vi "End Game.vi"(8 "error in (no error)":errorcluster, 11 "Game in":refnum<class "Game.lvclass">) -> (0 "error out":errorcluster, 3 "Game out":refnum<class "Game.lvclass">)   [LabVIEW 2020, in "SquareBattle.lvlib" / "Game.lvclass"]
uses:
  Game.lvclass
  Game.lvclass/Game.ctl
  Map/Map.lvclass
  Team/Team.lvclass
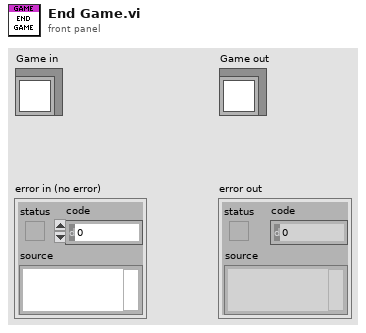
[diagram p1: front panel]
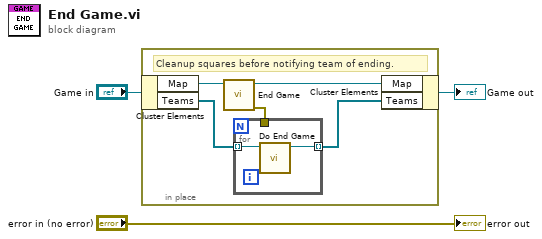
[diagram p0: block diagram]
diagram:
  n1 = in-place {
    # "Cleanup squares before notifying team of ending."
    n2 = in-place-cluster #1("Game in") -> ("Map"=w8:refnum<class "Map.lvclass">, "Teams"=w6:refnum<class "Team.lvclass">[])
    n3 = call "End Game.vi"("Map in"=w8) -> ("error out"=w4:errorcluster, "Map out"=w7:refnum<class "Map.lvclass">)  [unwired: 9 in]
    n4 = for {
      tunnel: w6 -> [w10] mode=indexing
      tunnel: [w9] -> w5 mode=indexing
      tunnel: w4 -> [_]
      n5 = call "Do End Game.vi"("Team in"=w10) -> ("Team out"=w9:refnum<class "Team.lvclass">)  [unwired: 10 in]
    }
    n6 = in-place-cluster #1("Map"=w7, "Teams"=w5) -> (→"Game out":refnum<class "Game.lvclass">)
  }
  "error out" <- "error in (no error)"
